vi "test-ElevatorSim-ALL-TESTS.vi"() -> (3 "All Passed":bool)   [LabVIEW 2019]
panel:
  out "Control Test":bool
  out "Min Max Test":bool
  out "Stability Test":bool
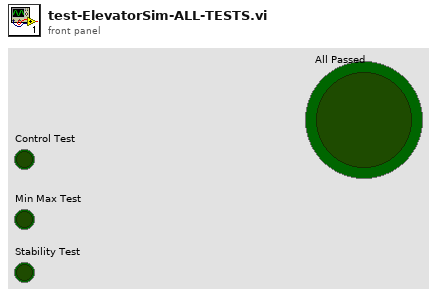
[diagram p1: front panel]
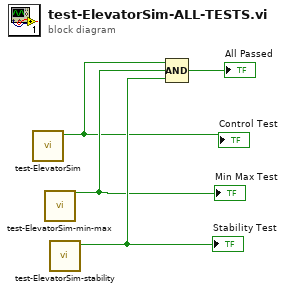
[diagram p0: block diagram]
diagram:
  n1 = call "test-ElevatorSim.vi"() -> ("Test Passed"=w1:bool)  [unwired: 11 in]
  "Control Test" <- w1
  n2 = call "test-ElevatorSim-min-max.vi"() -> ("Test Passed"=w2:bool)  [unwired: 11 in]
  "Min Max Test" <- w2
  n3 = call "test-ElevatorSim-stability.vi"() -> ("Test Passed"=w3:bool)  [unwired: 11 in]
  "Stability Test" <- w3
  n4 = Compound Arithmetic op=AND(w1, w2, w3) -> (→"All Passed":bool)
